vi "RegisterMap_ GenerateBase.vi"(11 "RegMap":T1[](array[typedef]) {"Mask" format="%.0x"}) -> (3 "Base Value":u16 format="%.0x")   [LabVIEW 2010]
uses:
  TYP_RegMap Item.ctl
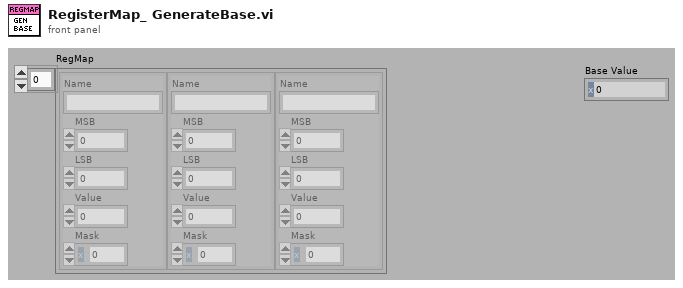
[diagram p1: front panel]
types:
  T1 = typedef "TYP_RegMap Item.ctl" = cluster{"Name":string, "MSB":u16, "LSB":u16, "Value":u16, "Mask":u16}
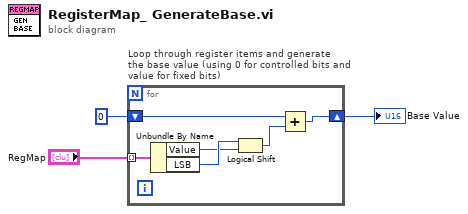
[diagram p0: block diagram]
diagram:
  n1 = for "Loop through register items and generate\nthe base value (using 0 for controlled bits and\nvalue for fixed bits)" {
    tunnel: "RegMap" -> [w8] mode=indexing
    shift-right: [w6] -> w2
    shift-left: u16 0 -> [w5]
    n2 = Unbundle By Name(w8) -> ("Value"=w7:u16, "LSB"=w9:u16)
    n3 = Logical Shift(y=w9, x=w7) -> (x << y=w4:u16)
    n4 = Add(x=w5, y=w4) -> (x+y=w6:u16)
  }
  "Base Value" <- w2
